vi "ContRunFPGA.vi"(3 "error in":errorcluster, 4 "Cluster":T1, 5 "runs slider ref":refnum<vi>, 6 "Line trig?":bool=TRUE) -> (0 "error out":errorcluster, 1 "times":u32[][](array[numeric]), 2 "readout":i16[][](array[numeric]))   [LabVIEW 2019]
uses:
  <vilib>/Utility/error.llb/Error Cluster From Error Code.vi
  <vilib>/rvi/errors/niLvFpgaAdjustHostInterfaceError.vi
  <vilib>/rvi/interface/nirviReadWriteControl/nirviReadWriteControl.xnode
  <vilib>/rvi/interface/nirviMethod/nirviMethod.xnode
  NiFpgaLv.dll
  <vilib>/rvi/interface/Simulation/niFpgaSimulationCallBeginRW.vi
  <vilib>/FPGAPlugInAG/Dynamic/niLvFpga_ReadFifo_Dynamic.vi
  <vilib>/rvi/errors/niLvFpgaMergeErrorWithErrorCode.vi
panel:
  out "stop graph":bool
  out "counts":cluster{u32[], u32[], u32[], u32[]}
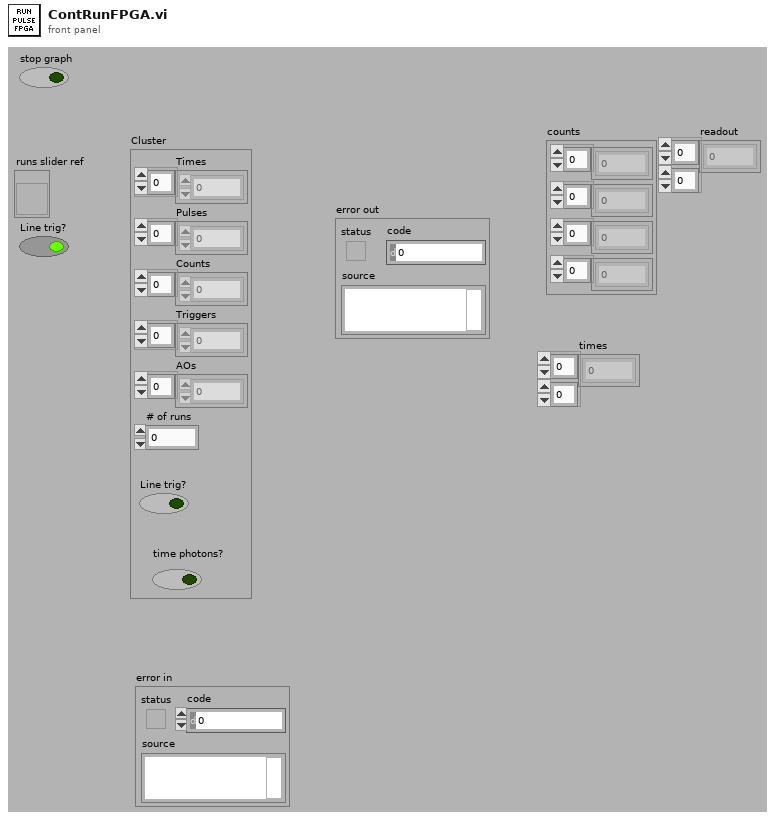
[diagram p1: front panel]
types:
  T1 = cluster{"Times":u32[], "Pulses":u64[], "Counts":u8[], "Triggers":u8[], "AOs":u8[], "# of runs":i32, "Line trig?":bool, "time photons?":bool}
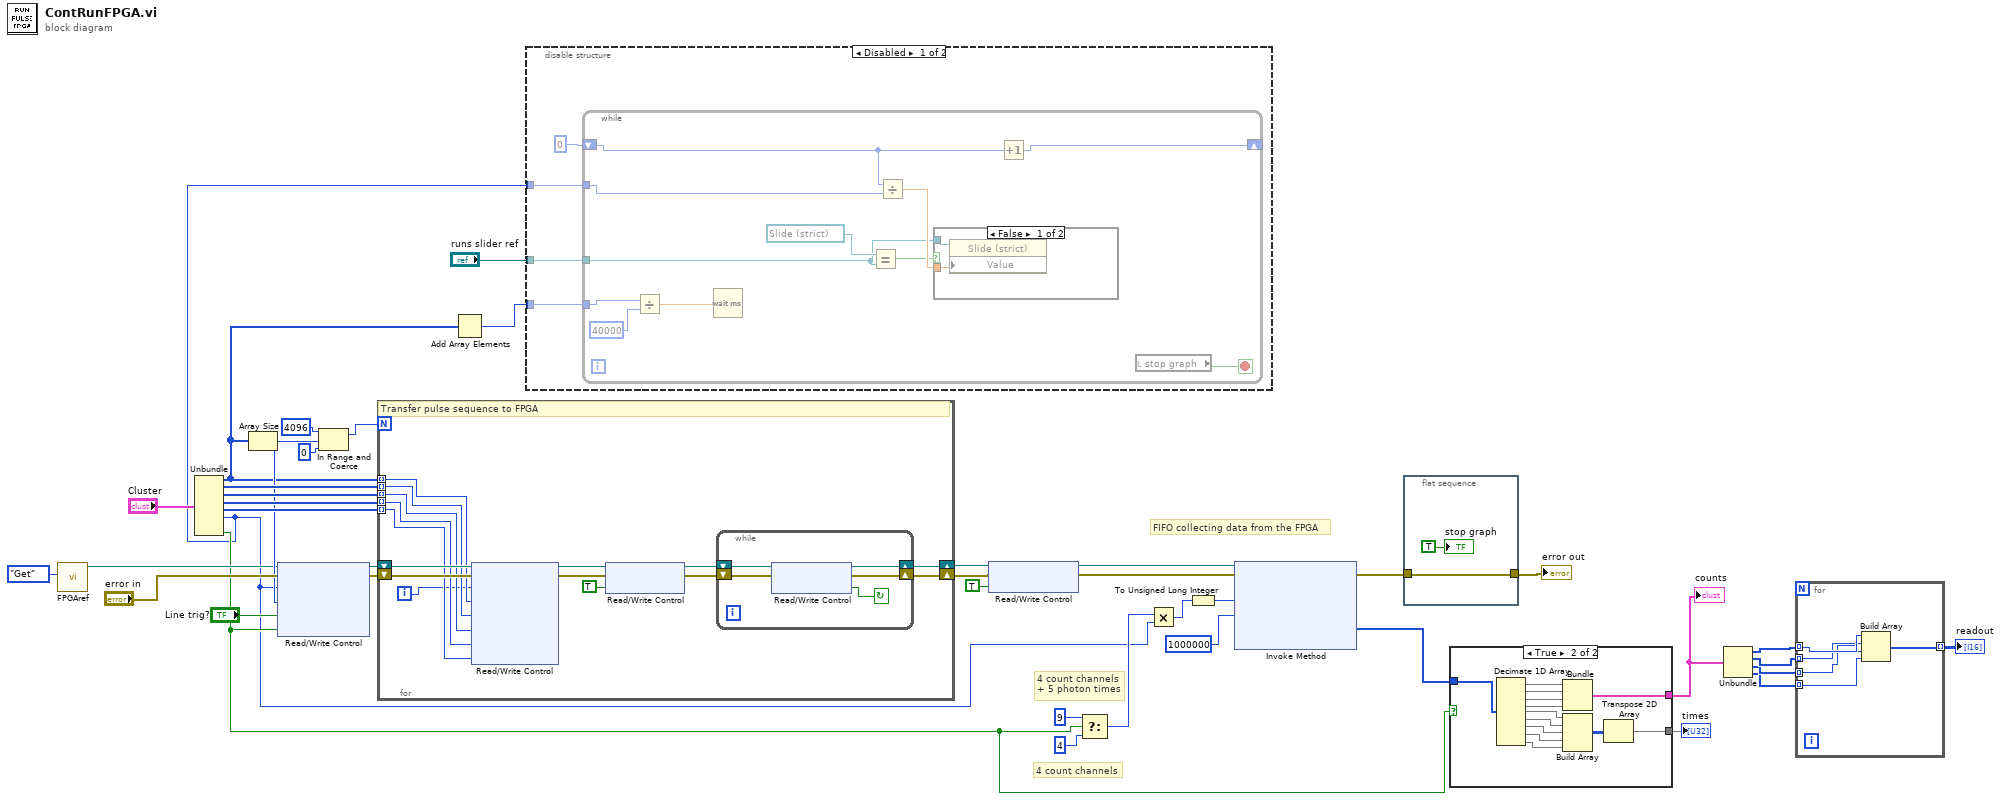
[diagram p0: block diagram]
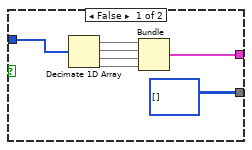
[diagram p4: hidden frame]
diagram:
  # "4 count channels\n+ 5 photon times"
  # "4 count channels"
  # "FIFO collecting data from the FPGA"
  n1 = call "FPGAref.vi"("Enum"=enum16{"Set", "Get"}."Get") -> ("FPGA VI Reference Out 2"=w22:refnum<k20>)  [unwired: 5 in, 1 out]
  n2 = Unbundle("Cluster") -> ("Times"=w1:u32[], "Pulses"=w35:u64[], "Counts"=w36:u8[], "Triggers"=w37:u8[], "AOs"=w38:u8[], "# of runs"=w2:i32, "time photons?"=w18:bool)  [unwired: 1 out]
  n3 = Array Size(array=w1) -> (size(s)=w23:i32)
  n4 = xnode "Read/Write Control"("FPGA VI Reference In"=w22, "error in"="error in", "# of runs"=w2, "# of pulses"=w23, "Line trig?"="Line trig?", "Send photons?"=w18) -> ("FPGA VI Reference Out"=w39:refnum<k20>, "error out"=w41:errorcluster)
  n5 = In Range and Coerce(upper limit=4096, x=w23, lower limit=0) -> (coerced(x)=w34:i32)  [unwired: 1 out]
  n6 = for {
    N: w34 -> [_]
    tunnel: w1 -> [w54] mode=indexing
    tunnel: w35 -> [w53] mode=indexing
    tunnel: w36 -> [w52] mode=indexing
    tunnel: w37 -> [w51] mode=indexing
    tunnel: w38 -> [w50] mode=indexing
    shift-right: [w44] -> w28
    shift-left: w39 -> [w56]
    shift-right: [w43] -> w29
    shift-left: w41 -> [w55]
    i -> [w42]
    # "Transfer pulse sequence to FPGA"
    n7 = xnode "Read/Write Control"("FPGA VI Reference In"=w56, "error in"=w55, "pulse number"=w42, "time data"=w54, "digout data"=w53, "count data"=w52, "trigger data"=w51, "AO data"=w50) -> ("FPGA VI Reference Out"=w48:refnum<k20>, "error out"=w47:errorcluster)
    n8 = xnode "Read/Write Control"("FPGA VI Reference In"=w48, "error in"=w47, "data waiting"=TRUE) -> ("FPGA VI Reference Out"=w46:refnum<k20>, "error out"=w45:errorcluster)
    n9 = while {
      shift-right: [w59] -> w44
      shift-left: w46 -> [w61]
      shift-right: [w58] -> w43
      shift-left: w45 -> [w60]
      stop <- w57 continue-if-true
      n10 = xnode "Read/Write Control"("FPGA VI Reference In"=w61, "error in"=w60) -> ("FPGA VI Reference Out"=w59:refnum<k20>, "error out"=w58:errorcluster, "data waiting"=w57:bool)
    }
  }
  n11 = Add Array Elements(numeric array=w1) -> (sum=w4:u32)
  n12 = disable-structure shown="Disabled" {
    disable-tunnel: w4 -> [w65 _]
    disable-tunnel: "runs slider ref" -> [w64 _]
    disable-tunnel: w2 -> [w62 _]
    frame Disabled {
      n13 = while {
        tunnel: w65 -> [w72]
        tunnel: w64 -> [w69]
        shift-right: [w68] -> _
        shift-left: 0 -> [w67]
        tunnel: w62 -> [w66]
        stop <- w73 stop-if-true
        n14 = Divide(x=w72, y=u32 40000) -> (x/y=w70:dbl)
        n15 = Wait (ms)(milliseconds to wait=w70) -> ()  [unwired: 1 out]
        n16 = Equal?(x=refnum<vi> refnum ("runs slider ref 2"), y=w69) -> (x = y?=w75:bool)
        n17 = Divide(x=w67, y=w66) -> (x/y=w76:dbl)
        n18 = case shown="False" w75 {
          tunnel: w76 -> [w78 _]
          tunnel: w69 -> [w77 _]
          frame False {
            n19 = property class="Slide (strict)"(reference=w77, "Value"=w78) -> ()  [unwired: 1 in, 2 out]
          }
          frame True {
          }
        }
        n20 = Increment(x=w67) -> (x+1=w68:i32)
        n21 = local read "stop graph"() -> (w73:bool)
      }
    }
    frame Enabled {
    }
  }
  n22 = xnode "Read/Write Control"("FPGA VI Reference In"=w28, "error in"=w29, "start sequence"=TRUE) -> ("FPGA VI Reference Out"=w24:refnum<k20>, "error out"=w25:errorcluster)
  n23 = Select(t=9, s=w18, f=4 ("x")) -> (s? t:f=w20:i32)
  n24 = Multiply(x=w20, y=w2) -> (x*y=w26:i32)
  n25 = To Unsigned Long Integer(number=w26) -> (unsigned 32bit integer=w27:u32)
  n26 = xnode "Invoke Method"("FPGA VI Reference In"=w24, "error in"=w25, "Number of Elements"=w27, "Timeout (ms)"=1000000) -> ("error out"=w6:errorcluster, "Data"=w17:u32[])  [unwired: 2 out]
  n27 = flat-sequence {
    tunnel: w6 -> [w80]
    tunnel: [w80] -> w5
    frame #0 {
      "stop graph" <- TRUE ("stop graph")
    }
  }
  n28 = case shown="True" w18 {
    tunnel: w17 -> [w87 w96]
    tunnel: [w82 w95] -> w14
    tunnel: [u32[][] [] ("transposed array") w88] -> w16
    frame False {
      n29 = Decimate 1D Array(w87) -> (w86:u32[], w85:u32[], w84:u32[], w83:u32[])
      n30 = Bundle(w86, w85, w84, w83) -> (w82:cluster{u32[], u32[], u32[], u32[]})  [unwired: 1 in]
    }
    frame True {
      n31 = Decimate 1D Array(w96) -> (w100:u32[], w99:u32[], w98:u32[], w97:u32[], w94:u32[], w93:u32[], w92:u32[], w91:u32[], w90:u32[])
      n32 = Bundle(w100, w99, w98, w97) -> (w95:cluster{u32[], u32[], u32[], u32[]})  [unwired: 1 in]
      n33 = Build Array(w94, w93, w92, w91, w90) -> (w89:u32[][])
      n34 = Transpose 2D Array(2D array=w89) -> (transposed array=w88:u32[][])
    }
  }
  "counts" <- w14
  "times" <- w16
  n35 = Unbundle(w14) -> (w13:u32[], w12:u32[], w11:u32[], w10:u32[])
  n36 = for {
    tunnel: w13 -> [w105] mode=indexing
    tunnel: w12 -> [w104] mode=indexing
    tunnel: w11 -> [w103] mode=indexing
    tunnel: w10 -> [w102] mode=indexing
    tunnel: [w101] -> w9 mode=indexing
    n37 = Build Array(w105, w104, w103, w102) -> (w101:u32[])
  }
  "readout" <- w9
  "error out" <- w5
